vi "Is Not Error.vi"(4 "enable (T)":bool=TRUE, 5 "error in":errorcluster) -> (0 "error out":errorcluster {"code" format="%.0x"}, 1 "ready":bool, 3 "!error":bool)   [LabVIEW 2020]
doc: "If Enabled is TRUE and !error is TRUE, then Ready is TRUE."
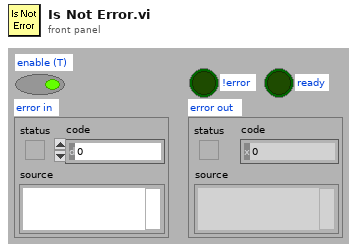
[diagram p1: front panel]
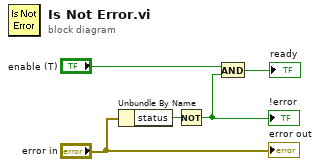
[diagram p0: block diagram]
diagram:
  n1 = Unbundle By Name("error in") -> ("status"=w4:bool)
  n2 = Not(x=w4) -> (.not. x?=w3:bool)
  "!error" <- w3
  n3 = And(x="enable (T)", y=w3) -> (x .and. y?=→"ready":bool)
  "error out" <- "error in"
